vi "DT_Triangle Manager_Add Edge_Double Side.vi"(4 "right bottom tri":i32, 5 "left bottom tri":i32, 6 "right top tri":i32, 7 "left top tri":i32, 8 "right point":i32, 9 "left point":i32, 10 "next triangle in":i32, 11 "Triangles In":i32[][](array[numeric])) -> (2 "next triangle out":i32, 3 "Triangles Out":i32[][](array[numeric]))   [LabVIEW 2017, in "NI_AAL_Geometry.lvlib"]
uses:
  <vilib>/Analysis/NI_AAL_Geometry.lvlib
  <vilib>/Analysis/geometry.llb/DT_Triangle Manager_Get Ghost Point.vi
  <vilib>/Analysis/geometry.llb/DT_Triangle Manager_Get Oppo Point.vi
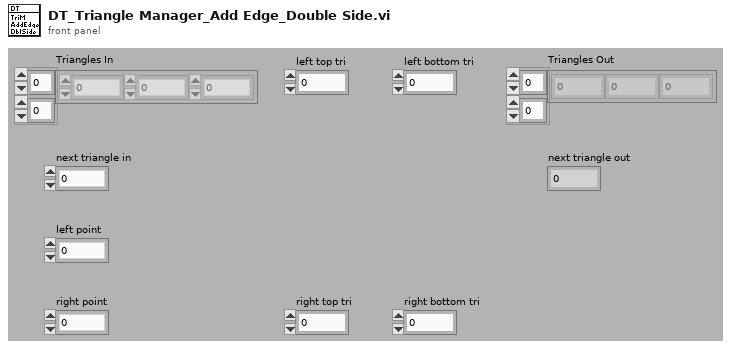
[diagram p1: front panel]
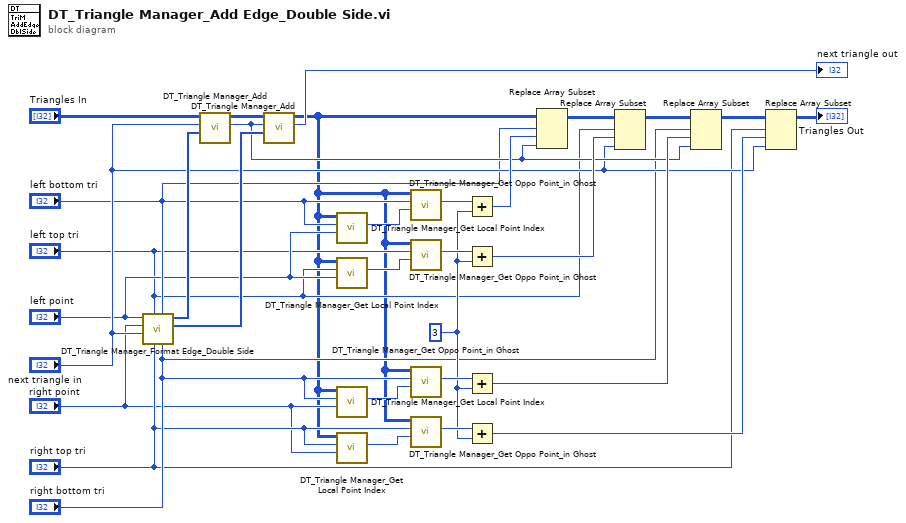
[diagram p0: block diagram]
diagram:
  w18 = 3 ("y")
  n1 = call <vilib>:"DT_Triangle Manager_Format Edge_Double Side.vi"("right bottom tri"="right bottom tri", "left bottom tri"="left bottom tri", "right top tri"="right top tri", "left top tri"="left top tri", "start triangle"="next triangle in", "right point"="right point", "left point"="left point") -> ("Second Triangle"=w28:i32[], "First Triangle"=w30:i32[])  [unwired: 3 out]
  n2 = call <vilib>:"DT_Triangle Manager_Add.vi"("Triangle"=w30, "next triangle in"="next triangle in", "Triangles In"="Triangles In") -> ("next triangle out"=w13:i32, "Triangles Out"=w31:i32[][])  [unwired: 7 out]
  n3 = call <vilib>:"DT_Triangle Manager_Add.vi"("Triangle"=w28, "next triangle in"=w13, "Triangles In"=w31) -> ("next triangle out"=→"next triangle out":i32, "Triangles Out"=w1:i32[][])  [unwired: 7 out]
  n4 = call <vilib>:"DT_Triangle Manager_Get Local Point Index.vi"("global idx"="left point", "triangle"="left bottom tri", "Triangles"=w1) -> ("local idx"=w10:i32)  [unwired: 8 out]
  n5 = call <vilib>:"DT_Triangle Manager_Get Local Point Index.vi"("global idx"="left point", "triangle"="left top tri", "Triangles"=w1) -> ("local idx"=w9:i32)  [unwired: 8 out]
  n6 = call <vilib>:"DT_Triangle Manager_Get Local Point Index.vi"("global idx"="right point", "triangle"="right bottom tri", "Triangles"=w1) -> ("local idx"=w5:i32)  [unwired: 8 out]
  n7 = call <vilib>:"DT_Triangle Manager_Get Local Point Index.vi"("global idx"="right point", "triangle"="right top tri", "Triangles"=w1) -> ("local idx"=w2:i32)  [unwired: 8 out]
  n8 = call <vilib>:"DT_Triangle Manager_Get Oppo Point_in Ghost.vi"("point idx"=w10, "triangle"="left bottom tri", "Triangles"=w1) -> ("opposite point idx"=w22:i32)  [unwired: 8 out]
  n9 = call <vilib>:"DT_Triangle Manager_Get Oppo Point_in Ghost.vi"("point idx"=w9, "triangle"="left top tri", "Triangles"=w1) -> ("opposite point idx"=w21:i32)  [unwired: 8 out]
  n10 = call <vilib>:"DT_Triangle Manager_Get Oppo Point_in Ghost.vi"("point idx"=w5, "triangle"="right bottom tri", "Triangles"=w1) -> ("opposite point idx"=w20:i32)  [unwired: 8 out]
  n11 = call <vilib>:"DT_Triangle Manager_Get Oppo Point_in Ghost.vi"("point idx"=w2, "triangle"="right top tri", "Triangles"=w1) -> ("opposite point idx"=w19:i32)  [unwired: 8 out]
  n12 = Add(x=w22, y=w18) -> (x+y=w17:i32)
  n13 = Add(x=w21, y=w18) -> (x+y=w16:i32)
  n14 = Add(x=w20, y=w18) -> (x+y=w15:i32)
  n15 = Add(x=w19, y=w18) -> (x+y=w14:i32)
  n16 = Replace Array Subset(array=w1, new element=w13, index (row)="left bottom tri", index (col)=w17) -> (w26:i32[][])
  n17 = Replace Array Subset(array=w26, new element="next triangle in", index (row)="left top tri", index (col)=w16) -> (w25:i32[][])
  n18 = Replace Array Subset(array=w25, new element=w13, index (row)="right bottom tri", index (col)=w15) -> (w24:i32[][])
  n19 = Replace Array Subset(array=w24, new element="next triangle in", index (row)="right top tri", index (col)=w14) -> (→"Triangles Out":i32[][])
